vi "PartB.vi"() -> ()   [LabVIEW 2010]
uses:
  <vilib>/Utility/file.llb/Write To Spreadsheet File (DBL).vi
  <vilib>/Analysis/NI_AALBase.lvlib
panel:
  out "Ampl":dbl
  in  "dfrequency":dbl format="%.2f"
  in  "Path":path
  in  "Slope":dbl
  in  "frequency":dbl format="%.2f"
  in  "ende":dbl
  in  "mode (0) 2":i16
  out "XY Graph":cluster{dbl[], dbl[]}(graph)
  out "error out 2":errorcluster
  in  "Wait/s":dbl format="%.2f"
  in  "Step":dbl format="%.2f"
  in  "mode (0)":i16
  in  "error in (no error)":errorcluster
  in  "Stop":dbl format="%.2f"
  in  "Starttemp":dbl format="%.2f"
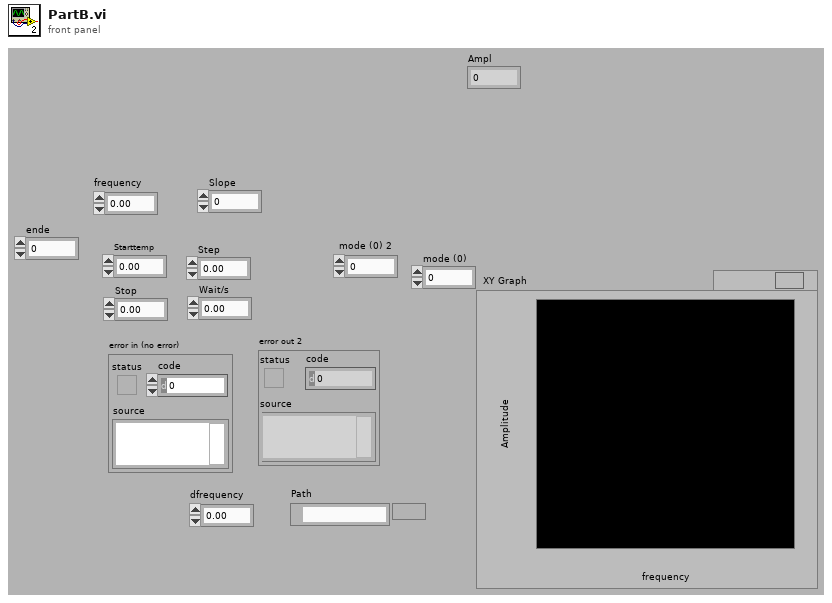
[diagram p1: front panel]
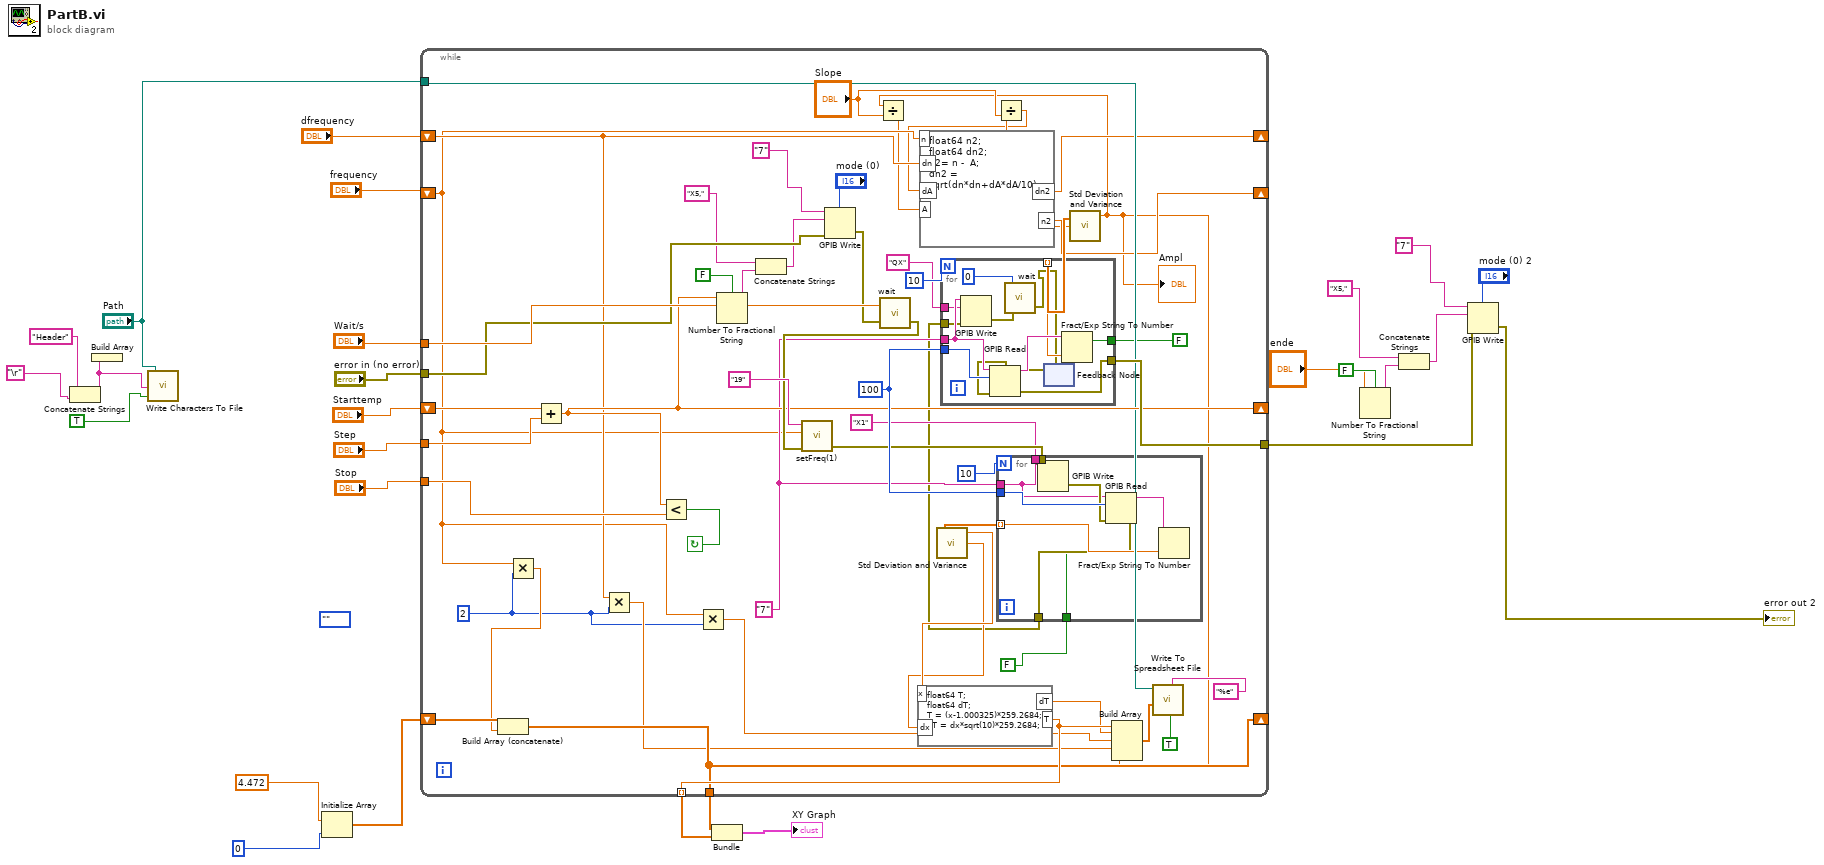
[diagram p0: block diagram]
diagram:
  (unwired) enum16{""}.""
  n1 = Concatenate Strings("Header", "\r") -> (w5:string)
  n2 = Build Array(w5) -> ()  [unwired: 1 out]
  n3 = call <vilib>:"Write Characters To File.vi"("append to file? (new file:F)"=TRUE, "character string"=w5, "file path (dialog if empty)"="Path") -> ()  [unwired: 2 in, 1 out]
  n4 = Initialize Array(4.472, 0) -> (w10:dbl[])
  n5 = while {
    tunnel: "error in (no error)" -> [w65]
    shift-right: [w60] -> _
    shift-left: "Starttemp" -> [w77]
    tunnel: "Step" -> [w79]
    tunnel: "Stop" -> [w78]
    tunnel: "Wait/s" -> [w75]
    tunnel: [w73] -> w2
    tunnel: [w51] -> w21 mode=indexing
    tunnel: [w45] -> w8
    shift-right: [w45] -> _
    shift-left: w10 -> [w61]
    shift-right: [w46] -> _
    shift-left: "frequency" -> [w33]
    tunnel: "Path" -> [w57]
    shift-right: [w47] -> _
    shift-left: "dfrequency" -> [w43]
    stop <- w76 continue-if-true
    w41 = 2
    w71 = 100
    w37 = "7"
    n6 = Multiply(x=w33, y=w41) -> (x*y=w44:dbl)
    n7 = Build Array (concatenate)(w61, w44) -> (w45:dbl[])
    n8 = Add(x=w77, y=w79) -> (x+y=w60:dbl)
    n9 = Multiply(x=w43, y=w41) -> (x*y=w42:dbl)
    n10 = Less?(x=w60, y=w78) -> (x < y?=w76:bool)
    n11 = Multiply(x=w33, y=w41) -> (x*y=w40:dbl)
    n12 = Number To Fractional String(use system decimal point (T)=FALSE, number=w60) -> (F-format string=w64:string)  [unwired: 2 in]
    n13 = Concatenate Strings("X5,", w64) -> (w62:string)
    n14 = GPIB Write(0:"7", 1:w62, 2:"mode (0)", 3:w65) -> (6:w67:errorcluster)  [unwired: 1 in, 1 out]
    n15 = call "wait.vi"("error in"=w67, "Wartezeit in Sek"=w75) -> ("error out"=w66:errorcluster)  [unwired: 1 in]
    n16 = call "setFreq(1).vi"("error in"=w66, "Frequenz in Hz"=w33, "address string"="19") -> ("error out"=w39:errorcluster)  [unwired: 3 in]
    n17 = for {
      N: 10 -> [_]
      tunnel: w37 -> [w95]
      tunnel: FALSE -> [w92]
      tunnel: w71 -> [w100]
      tunnel: [w99] -> w54 mode=indexing
      tunnel: [w97] -> w35
      tunnel: w39 -> [w94]
      tunnel: "X1" -> [w93]
      n18 = GPIB Write(0:w95, 1:w93, 3:w94) -> (6:w96:errorcluster)  [unwired: 2 in, 1 out]
      n19 = GPIB Read(0:w95, 1:w100, 3:w96) -> (5:w98:string, 7:w97:errorcluster)  [unwired: 2 in, 1 out]
      n20 = Fract/Exp String To Number(use system decimal point (T)=w92, string=w98) -> (number=w99:dbl)  [unwired: 2 in, 1 out]
    }
    n21 = call <vilib>:"Std Deviation and Variance.vi"("X"=w54) -> ("mean"=w53:dbl, "standard deviation"=w52:dbl)  [unwired: 1 in, 1 out]
    n22 = formula code="float64 T;\nfloat64 dT;\nT = (x-1.000325)*259.2684;\ndT = dx*sqrt(10)*259.2684;"("x"=w53, "dx"=w52) -> ("T"=w51:dbl, "dT"=w50:dbl)
    n23 = for {
      N: 10 -> [_]
      tunnel: [w91] -> w73
      tunnel: w37 -> [w88]
      tunnel: w71 -> [w90]
      tunnel: [w84] -> w48 mode=indexing
      tunnel: "QX" -> [w87]
      tunnel: w35 -> [w86]
      tunnel: FALSE ("use system decimal point (T)") -> [w85]
      n24 = GPIB Write(0:w88, 1:w87, 3:w86) -> (6:w83:errorcluster)  [unwired: 2 in, 1 out]
      n25 = call "wait.vi"("error in"=w83, "Wartezeit in Sek"=0) -> ("error out"=w82:errorcluster)  [unwired: 1 in]
      n26 = feedback-in #1(w82) -> ()
      n27 = feedback #1() -> (w81:errorcluster)  [unwired: 1 in]
      n28 = GPIB Read(0:w88, 1:w90, 3:w81) -> (5:w89:string, 7:w91:errorcluster)  [unwired: 2 in, 1 out]
      n29 = Fract/Exp String To Number(use system decimal point (T)=w85, string=w89) -> (number=w84:dbl)  [unwired: 2 in, 1 out]
    }
    n30 = call <vilib>:"Std Deviation and Variance.vi"("X"=w48) -> ("mean"=w28:dbl, "standard deviation"=w30:dbl)  [unwired: 1 in, 1 out]
    "Ampl" <- w28
    n31 = Divide(x=w28, y="Slope") -> (x/y=w32:dbl)
    n32 = Divide(x=w30, y="Slope") -> (x/y=w29:dbl)
    n33 = formula code="float64 n2;\nfloat64 dn2;\nn2= n -  A;\ndn2 = sqrt(dn*dn+dA*dA/10);"("n"=w33, "A"=w32, "dA"=w29, "dn"=w43) -> ("n2"=w46:dbl, "dn2"=w47:dbl)
    n34 = Build Array(w51, w50, w40, w42, w28) -> (w56:dbl[])
    n35 = call-poly <vilib>:"Write To Spreadsheet File.vi"("format (%.3f)"="%e", "append to file? (new file:F)"=TRUE, "1D data"=w56, "file path (dialog if empty)"=w57) -> ()  [unwired: 4 in, 1 out]
  }
  n36 = Bundle(w8, w21) -> (→"XY Graph":cluster{dbl[], dbl[]})  [unwired: 1 in]
  n37 = Number To Fractional String(use system decimal point (T)=FALSE, number="ende") -> (F-format string=w17:string)  [unwired: 2 in]
  n38 = Concatenate Strings("X5,", w17) -> (w15:string)
  n39 = GPIB Write(0:"7", 1:w15, 2:"mode (0) 2", 3:w2) -> (6:→"error out 2":errorcluster)  [unwired: 1 in, 1 out]
